vi "Main VI.vi"(8 "error in (no error)":errorcluster, 11 "FPGA VI Reference In":refnum<k20>) -> (0 "error out":errorcluster)   [LabVIEW 2023, in "FPGA.lvlib"]
uses:
  FPGA.lvlib
  Internal Communication/Internal Communication.lvlib
  <vilib>/rvi/interface/nirviCloseFPGA/nirviCloseFPGA.xnode
  <vilib>/FPGAPlugInAG/Dynamic/niLvFpga_Close_Dynamic.vi
  Encoder/Encoder.lvlib
panel:
  in  "stop":bool
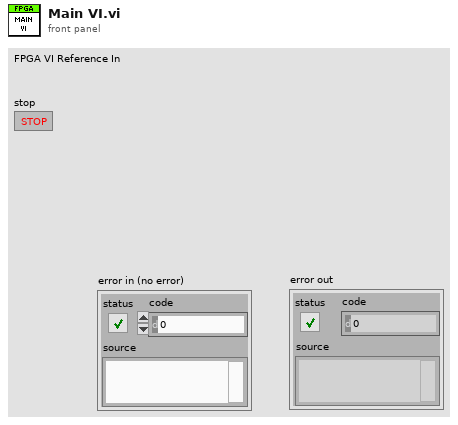
[diagram p1: front panel]
types:
  T1 = typedef "Queue.ctl" = refnum<queue>
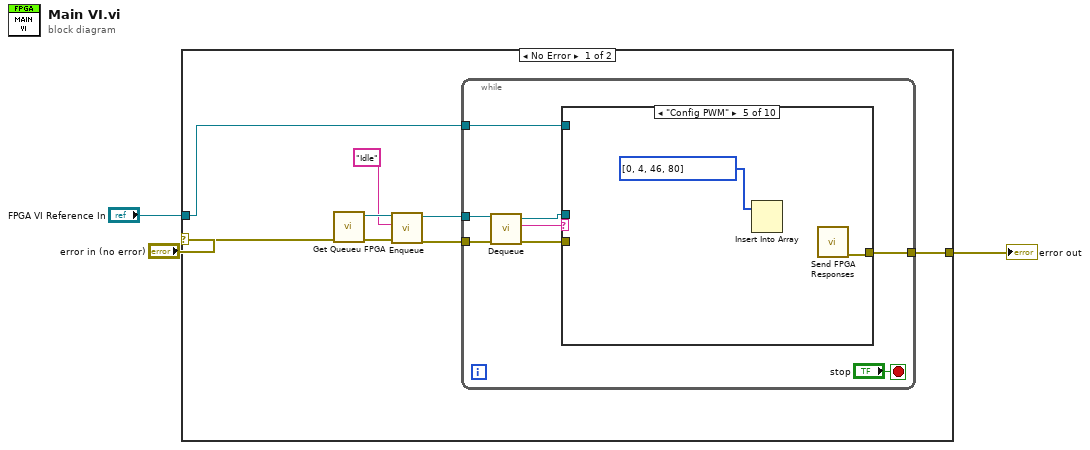
[diagram p0: block diagram]
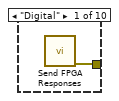
[diagram p2: hidden frame]
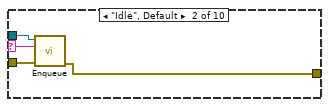
[diagram p3: hidden frame]
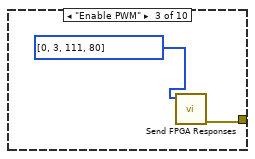
[diagram p4: hidden frame]
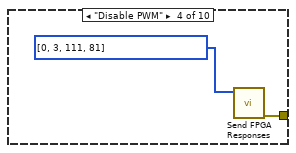
[diagram p5: hidden frame]
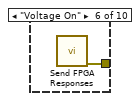
[diagram p6: hidden frame]
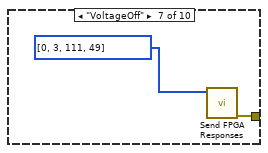
[diagram p7: hidden frame]
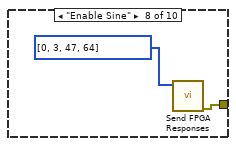
[diagram p8: hidden frame]
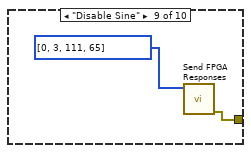
[diagram p9: hidden frame]
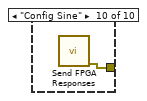
[diagram p10: hidden frame]
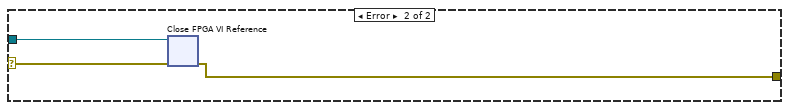
[diagram p11: hidden frame]
diagram:
  n1 = case shown="No Error" "error in (no error)" {
    selector: "error in (no error)" -> [w11 w41]
    tunnel: [w5 w39] -> w2
    tunnel: "FPGA VI Reference In" -> [w4 w40]
    frame No Error {
      n2 = call "Get Queueu FPGA.vi"("error in (no error)"=w11) -> ("error out"=w10:errorcluster, "Error Queue"=w9:refnum<queue>)  [unwired: 9 in]
      n3 = call "Enqueue.vi"("error in (no error)"=w10, "Command"="Idle", "Queue In"=w9) -> ("error out"=w7:errorcluster, "Queue Out"=w6:T1)  [unwired: 7 in]
      n4 = while {
        tunnel: w7 -> [w19]
        tunnel: w6 -> [w18]
        tunnel: [w14] -> w5
        tunnel: w4 -> [w12]
        stop <- "stop" stop-if-true
        n5 = call "Dequeue.vi"("error in (no error)"=w19, "Queue In"=w18) -> ("error out"=w16:errorcluster, "String"=w17:string, "Queue Out"=w15:T1)  [unwired: 6 in, 1 out]
        n6 = case shown="\"Config PWM\"" w17 {
          selector: w17 -> [_ w22 _ _ _ _ _ _ _ _]
          tunnel: w16 -> [_ w24 _ _ _ _ _ _ _ _]
          tunnel: w15 -> [_ w23 _ _ _ _ _ _ _ _]
          tunnel: [w20 w21 w26 w28 w30 w31 w33 w35 w37 w38] -> w14
          tunnel: w12 -> [_ _ _ _ _ _ _ _ _ _]
          frame "Digital" {
            n7 = call "Send FPGA Responses.vi"() -> ("error out"=w20:errorcluster)  [unwired: 11 in]
          }
          frame "Idle", Default {
            n8 = call "Enqueue.vi"("error in (no error)"=w24, "Command"=w22, "Queue In"=w23) -> ("error out"=w21:errorcluster)  [unwired: 7 in, 1 out]
          }
          frame "Enable PWM" {
            n9 = call "Send FPGA Responses.vi"("Data"=u8[] [0, 3, 111, 80] ("Array")) -> ("error out"=w26:errorcluster)  [unwired: 10 in]
          }
          frame "Disable PWM" {
            n10 = call "Send FPGA Responses.vi"("Data"=u8[] [0, 3, 111, 81] ("Array")) -> ("error out"=w28:errorcluster)  [unwired: 10 in]
          }
          frame "Config PWM" {
            n11 = Insert Into Array(array=u8[] [0, 4, 46, 80] ("Array")) -> ()  [unwired: 2 in, 1 out]
            n12 = call "Send FPGA Responses.vi"() -> ("error out"=w30:errorcluster)  [unwired: 11 in]
          }
          frame "Voltage On" {
            n13 = call "Send FPGA Responses.vi"() -> ("error out"=w31:errorcluster)  [unwired: 11 in]
          }
          frame "VoltageOff" {
            n14 = call "Send FPGA Responses.vi"("Data"=u8[] [0, 3, 111, 49] ("Array")) -> ("error out"=w33:errorcluster)  [unwired: 10 in]
          }
          frame "Enable Sine" {
            n15 = call "Send FPGA Responses.vi"("Data"=u8[] [0, 3, 47, 64] ("Array")) -> ("error out"=w35:errorcluster)  [unwired: 10 in]
          }
          frame "Disable Sine" {
            n16 = call "Send FPGA Responses.vi"("Data"=u8[] [0, 3, 111, 65] ("Array")) -> ("error out"=w37:errorcluster)  [unwired: 10 in]
          }
          frame "Config Sine" {
            n17 = call "Send FPGA Responses.vi"() -> ("error out"=w38:errorcluster)  [unwired: 11 in]
          }
        }
      }
    }
    frame Error {
      n18 = xnode "Close FPGA VI Reference"("FPGA VI Reference In"=w40, "error in"=w41) -> ("error out"=w39:errorcluster)
    }
  }
  "error out" <- w2
